vi "gh-cli Release Upload.vi"(8 "error in (no error)":errorcluster, 10 "Options":string, 11 "Git in":refnum<class "Git.lvclass">) -> (0 "error out":errorcluster, 2 "standard output":string, 3 "Git out":refnum<class "Git.lvclass">)   [LabVIEW 2019, in "Git.lvclass"]
doc: "gh release upload <tag> <files>... [flags]: Upload asset files to a GitHub Release.\n\nTo define a display label for an asset, append text starting with '#' after the file name.\n\n<b>Options</b>\n--clobber Overwrite existing as sets of the same name\n-R, --repo <[HOST/]OWNER/REPO>: Select another repository using the [HOST/]OWNER/REPO format \n\nhttps://cli.github.com/manual"
uses:
  Git.lvclass
  Git.lvclass/Git.ctl
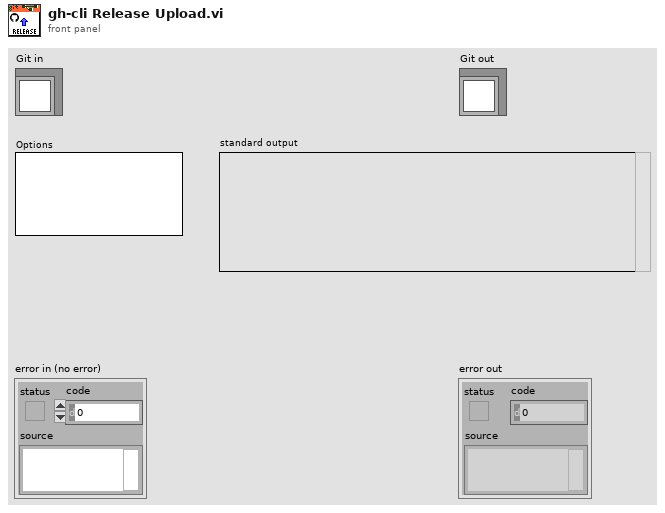
[diagram p1: front panel]
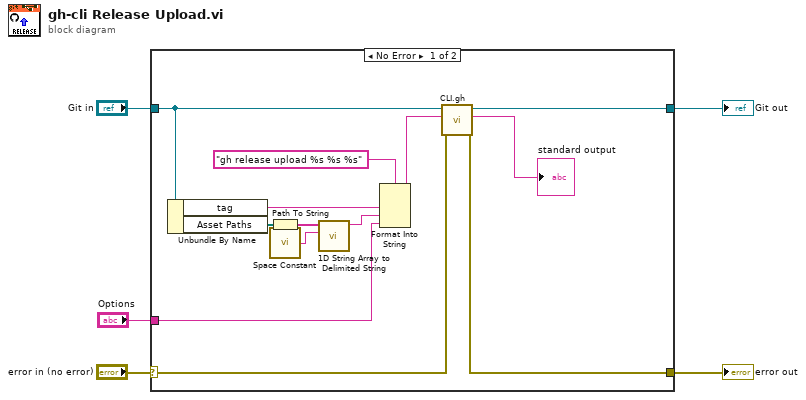
[diagram p0: block diagram]
diagram:
  n1 = case shown="No Error" "error in (no error)" {
    selector: "error in (no error)" -> [w17 w20]
    tunnel: [w16 w20] -> w4
    tunnel: [w18 w19] -> w2
    tunnel: "Git in" -> [w13 w19]
    tunnel: "Options" -> [w7 _]
    frame No Error {
      n2 = Unbundle By Name(w13) -> ("tag"=w12:string, "Asset Paths"=w11:path[])
      n3 = Path To String(path=w11) -> (string=w10:string[])
      n4 = call <vilib>:"Space Constant.vi"() -> ("String"=w8:string)
      n5 = call <vilib>:"1D String Array to Delimited String.vi"("delimiter"=w8, "string array"=w10) -> ("delimited string"=w9:string)  [unwired: 9 in]
      n6 = Format Into String(format string="gh release upload %s %s %s", w12, w9, w7) -> (resulting string=w6:string)  [unwired: 2 in, 1 out]
      n7 = call "CLI.gh.vi"("error in (no error)"=w17, "Command"=w6, "Git in"=w13) -> ("error out"=w16:errorcluster, "standard output"=→"standard output":string, "Git out"=w18:refnum<class "Git.lvclass">)  [unwired: 4 in, 2 out]
    }
    frame Error {
    }
  }
  "error out" <- w4
  "Git out" <- w2
